vi "FPGA_Code_Dummy.vi"() -> ()   [LabVIEW 2018]
uses:
  <vilib>/rvi/eio/common/nirviEmuTemplateMethod_errors.vi
  <vilib>/eio/EIONode/EIONode.xnode
panel:
  out "BooleanLEDInFPGACode":bool
  in  "BooleanButtonInFPGACode":bool
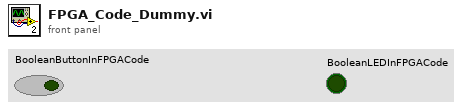
[diagram p1: front panel]
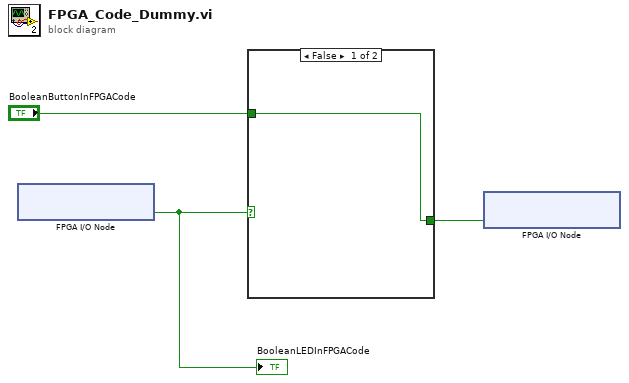
[diagram p0: block diagram]
diagram:
  n1 = xnode "FPGA I/O Node"() -> ("Connector0/DIO0"=w1:bool)  [unwired: 1 in, 1 out]
  "BooleanLEDInFPGACode" <- w1
  n2 = case shown="False" w1 {
    tunnel: "BooleanButtonInFPGACode" -> [w4 w5]
    tunnel: [w4 w5] -> w2
    frame False {
    }
    frame True {
    }
  }
  n3 = xnode "FPGA I/O Node"("Connector0/DIO1"=w2) -> ()  [unwired: 1 in, 1 out]
